vi "Configure.vi"(8 "error in (no error)":errorcluster, 10 "ConfigRef In":T1, 11 "Yokogawa in":refnum<class "Yokogawa.lvclass">) -> (0 "error out":errorcluster, 3 "Yokogawa out":refnum<class "Yokogawa.lvclass">)   [LabVIEW 2015, in "Yokogawa.lvclass"]
uses:
  Yokogawa.lvclass
  <vilib>/Utility/config.llb/Config Data RefNum.ctl
  Parent/Power Meter.lvclass/Power Meter.ctl
  Parent/Write Address.vi
  <vilib>/Utility/config.llb/Read Key (String).vi
  <vilib>/Utility/config.llb/Read Key (Double).vi
  <vilib>/Utility/config.llb/NI_LVConfig.lvlib
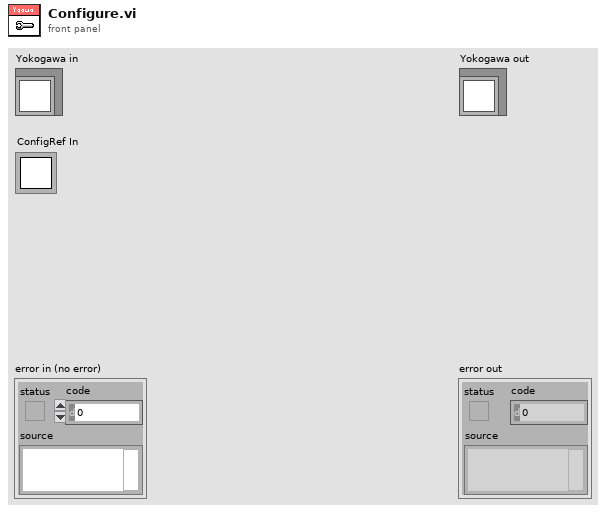
[diagram p1: front panel]
types:
  T1 = typedef "NI_LVConfig.lvlib/Config Data RefNum.ctl" = refnum<k1>
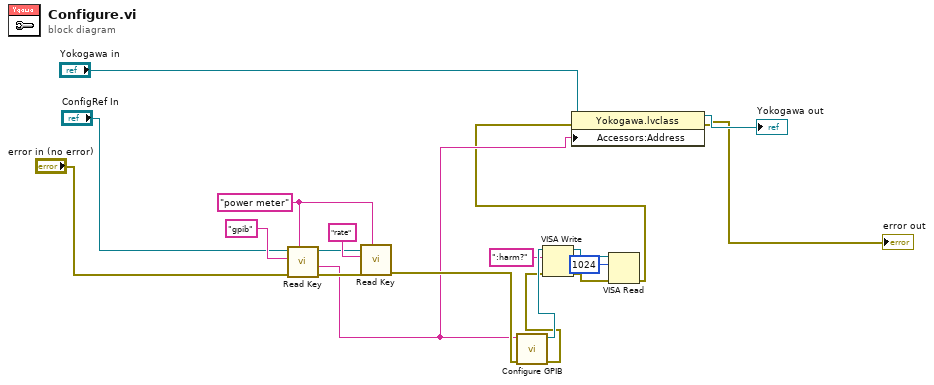
[diagram p0: block diagram]
diagram:
  w18 = "power meter" ("section")
  n1 = call-poly <vilib>:"Read Key.vi"("section"=w18, "error in (no error)"="error in (no error)", "key"="gpib", "refnum"="ConfigRef In") -> ("error out"=w17:errorcluster, "value"=w5:string, "refnum out"=w16:T1)  [unwired: 4 in, 1 out]
  n2 = call-poly <vilib>:"Read Key.vi"("section"=w18, "error in (no error)"=w17, "key"="rate", "refnum"=w16) -> ("error out"=w14:errorcluster)  [unwired: 4 in, 3 out]
  n3 = call "Configure GPIB.vi"("error in"=w14, "VISA Refnum in"=w5) -> ("error out"=w3:errorcluster, "VISA resource name out"=w13:refnum<visa-resource-name>)  [unwired: 8 in]
  n4 = VISA Write(VISA resource name=w13, write buffer=":harm?", error in (no error)=w3) -> (VISA resource name out=w11:refnum<visa-resource-name>, error out=w10:errorcluster)  [unwired: 1 out]
  n5 = VISA Read(VISA resource name=w11, byte count=u32 1024, error in (no error)=w10) -> (error out=w2:errorcluster)  [unwired: 3 out]
  n6 = property class="Yokogawa.lvclass"(reference="Yokogawa in", error in=w2, "Accessors:Address"=w5) -> (reference out=→"Yokogawa out":refnum<class "Yokogawa.lvclass">, error out=→"error out":errorcluster)
